vi "Capture UI State.vi"(5 "Ctls Refs (All Ctls)":refnum<vi>[](array[refnum]), 6 "Traverse Clusters (F)":bool, 7 "VI Ref (Calling VI)":refnum<vi>, 8 "Error In":errorcluster, 10 "State Name":string, 11 "UIM In":refnum<data-value>) -> (0 "Error Out":errorcluster, 3 "UIM Out":refnum<data-value>)   [LabVIEW 2020, in "UIM.lvlib" / "UIM.lvclass"]
doc: "Capture a VIs current state under a name you specify at the input. You can refer to that name when restoring or removing that state. If the name existed before it will be overwritten.\n\n<b>VI Ref (Calling VI) -</b> Allows you to point to the VI you want to work with. If the VI Ref is left unwired the calling VI reference will be used. \n\n<b>Ctls Refs (All Ctls) -</b> If the Ctls Refs are unwired, all control references and their properties, handled by UIPs in the UIM, will be captured to the state definition. By wiring this input you can optimize the performance of this method, because it will not need to traverse and obtain references to all controls and indicators of a VIs front panel.\n\n<b>Travers Clusters -</b> Defines if the clusters are considered compound controls, disposing their contents, or not. Use this if you want to capture the UIPs on the controls inside of clusters."
uses:
  UIM.lvclass
  UIM.lvclass/UIM.ctl
  UIP Interface/UIP Interface.lvclass
  <vilib>/Utility/LVClass/Get LV Class Name.vi
  <vilib>/Utility/error.llb/Error Cluster From Error Code.vi
  <vilib>/ErrorRing/Error Ring.xnode
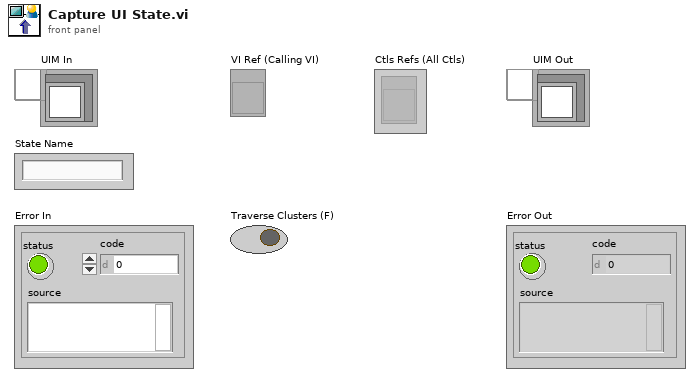
[diagram p1: front panel]
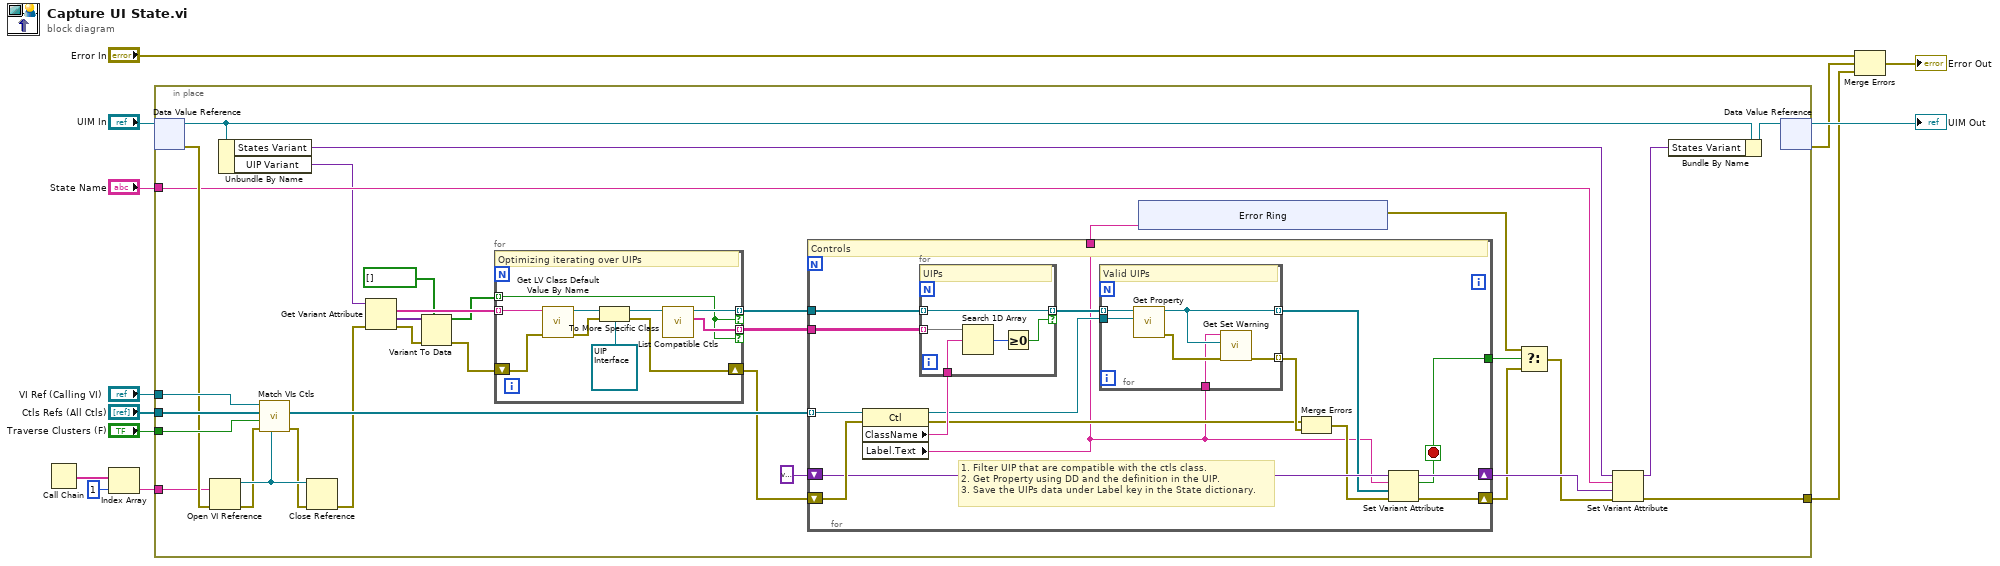
[diagram p0: block diagram]
diagram:
  n1 = Call Chain() -> (call chain=w2:string[])
  n2 = Index Array(array=w2, index=1) -> (element=w1:string)
  n3 = in-place {
    in-place-border: "VI Ref (Calling VI)" -> [w46]
    in-place-border: "Ctls Refs (All Ctls)" -> [w45]
    in-place-border: "State Name" -> [w35]
    in-place-border: "Traverse Clusters (F)" -> [w38]
    in-place-border: [w33] -> w4
    in-place-border: w1 -> [w19]
    n4 = in-place-dvr #1("UIM In") -> (w32:refnum<class "UIM.lvclass">, w37:errorcluster)
    n5 = Open VI Reference(vi path=w19, error in (no error)=w37) -> (vi reference=w43:refnum<vi>, error out=w41:errorcluster)  [unwired: 4 out]
    n6 = Unbundle By Name(w32) -> ("States Variant"=w36:variant, "UIP Variant"=w27:variant)
    n7 = call "Match VIs Ctls.vi"("Calling VI Ref"=w43, "Error In"=w41, "Traverse Clusters (F)"=w38, "Ctls Refs (All Ctls)"=w45, "VI Ref"=w46) -> ("Error Out"=w42:errorcluster, "Matching Ctls Out"=w44:refnum<vi>[])  [unwired: 4 in, 1 out]
    n8 = Close Reference(reference=w43, error in (no error)=w42) -> (error out=w20:errorcluster)
    n9 = Get Variant Attribute(Variant=w27, error in=w20) -> (names=w26:string[], values=w24:variant[], error out=w22:errorcluster)  [unwired: 2 in, 1 out]
    n10 = Variant To Data(error in=w22, type=bool[] [], Variant=w24) -> (data=w21:bool[], error out=w23:errorcluster)
    n11 = for {
      tunnel: [w63] -> w40 mode=indexing if=w55
      tunnel: [w62] -> w39 mode=indexing if=w55
      tunnel: w26 -> [w61] mode=indexing
      shift-right: [w56] -> w28
      shift-left: w23 -> [w54]
      tunnel: w21 -> [w55] mode=indexing
      # "Optimizing iterating over UIPs"
      n12 = call <vilib>:"Get LV Class Default Value By Name.vi"("error in (no error)"=w54, "class name"=w61) -> ("error out"=w57:errorcluster, "object"=w60:refnum<class>)  [unwired: 8 in]
      n13 = To More Specific Class(target class=refnum<class "UIP Interface.lvclass"> refnum ("UIP In"), reference=w60, error in=w57) -> (specific class reference=w58:refnum<class "UIP Interface.lvclass">, error out=w56:errorcluster)
      n14 = call-dynamic "List Compatible Ctls.vi"("UIP In"=w58) -> ("Compatible Ctl Classes"=w62:string[], "UIP Out"=w63:refnum<class "UIP Interface.lvclass">)  [unwired: 9 in]
    }
    n15 = for {
      tunnel: w44 -> [w79] mode=indexing
      shift-right: [w68] -> w17
      shift-left: w28 -> [w75]
      shift-right: [w69] -> w34
      shift-left: variant -> [w71]
      tunnel: w40 -> [w74]
      tunnel: w39 -> [w73]
      tunnel: [w65] -> w15
      tunnel: [w64] -> w18
      stop <- w64 stop-if-true
      # "1. Filter UIP that are compatible with the ctls class.\n2. Get Property using DD and the definition in the UIP.\n3. Save the UIPs data under Label key in the State dictionary."
      # "Controls"
      n16 = property class="Ctl"(reference=w79, error in=w75) -> (reference out=w76:refnum<vi>, error out=w67:errorcluster, "ClassName"=w78:string, "Label.Text"=w65:string)
      n17 = for {
        tunnel: [w87] -> w77 mode=indexing if=w89
        tunnel: w78 -> [w88]
        tunnel: w74 -> [w87] mode=indexing
        tunnel: w73 -> [w86] mode=indexing
        # "UIPs"
        n18 = Search 1D Array(1D array=w86, element=w88) -> (index of element=w90:i32)  [unwired: 1 in]
        n19 = Greater Or Equal To 0?(x=w90) -> (x >= 0?=w89:bool)
      }
      n20 = for {
        tunnel: w77 -> [w85] mode=indexing
        tunnel: w76 -> [w84]
        tunnel: [w83] -> w70 mode=indexing
        tunnel: [w81] -> w72 mode=indexing
        tunnel: w65 -> [w80]
        # "Valid UIPs"
        n21 = call-dynamic "Get Property.vi"("Ctl Ref"=w84, "UIP In"=w85) -> ("Error Out"=w82:errorcluster, "UIP Out"=w83:refnum<class "UIP Interface.lvclass">)  [unwired: 8 in]
        n22 = call "Get Set Warning.vi"("Error In"=w82, "UIP"=w83, "Label.Text"=w80) -> ("Error Out"=w81:errorcluster)  [unwired: 8 in]
      }
      n23 = Merge Errors(w67, w72) -> (w66:errorcluster)
      n24 = Set Variant Attribute(Variant=w71, name=w65, value=w70, error in=w66) -> (Variant out=w69:variant, replaced=w64:bool, error out=w68:errorcluster)
    }
    n25 = xnode "Error Ring"("parameter 0"=w15) -> ("error out"=w14:errorcluster)
    n26 = Select(t=w14, s=w18, f=w17) -> (s? t:f=w16:errorcluster)
    n27 = Set Variant Attribute(Variant=w36, name=w35, value=w34, error in=w16) -> (Variant out=w30:variant, error out=w33:errorcluster)  [unwired: 1 out]
    n28 = Bundle By Name(cluster=w32, "States Variant"=w30) -> (w31:refnum<class "UIM.lvclass">)
    n29 = in-place-dvr #1(w31) -> (→"UIM Out":refnum<data-value>, w5:errorcluster)
  }
  n30 = Merge Errors("Error In", w5, w4) -> (→"Error Out":errorcluster)
